vi "test-SyncMessageInCSMF.vi"(8 "error in (no error)":errorcluster, 11 "TestCase in":refnum<class "testcase-CSMSyncMessage.lvclass">) -> (0 "error out":errorcluster, 3 "TestCase out":refnum<class "testcase-CSMSyncMessage.lvclass">)   [LabVIEW 2017, in "testcase-CSMSyncMessage.lvclass"]
uses:
  testcase-CSMSyncMessage.lvclass
  src/user.lib/_NEVSTOP/Communicable State Machine(CSM)/AdvanceAPI/CSM - Make String Arguments Safe.vi
  src/user.lib/_NEVSTOP/Communicable State Machine(CSM)/AdvanceAPI/CSM - Keywords.vi
  CSM/Global-TestcaseCSM.vi
  <vilib>/addons/_JKI Toolkits/VI Tester/TestCase.llb/TestCase.lvclass
  src/user.lib/_NEVSTOP/Communicable State Machine(CSM)/Communicable State Machine.lvlib
  C:/Program Files (x86)/National Instruments/LabVIEW 2017/vi.lib/addons/_JKI Toolkits/VI Tester/TestCase.llb/TestCase.lvclass
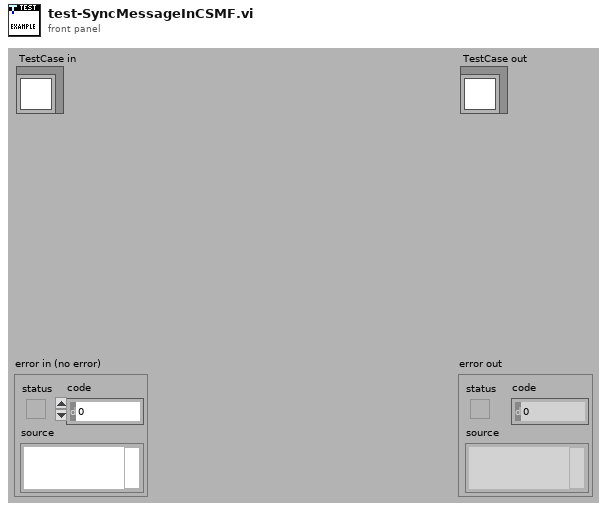
[diagram p1: front panel]
types:
  T1 = cluster{"Arguments":string, "Response":string, "error":errorcluster}
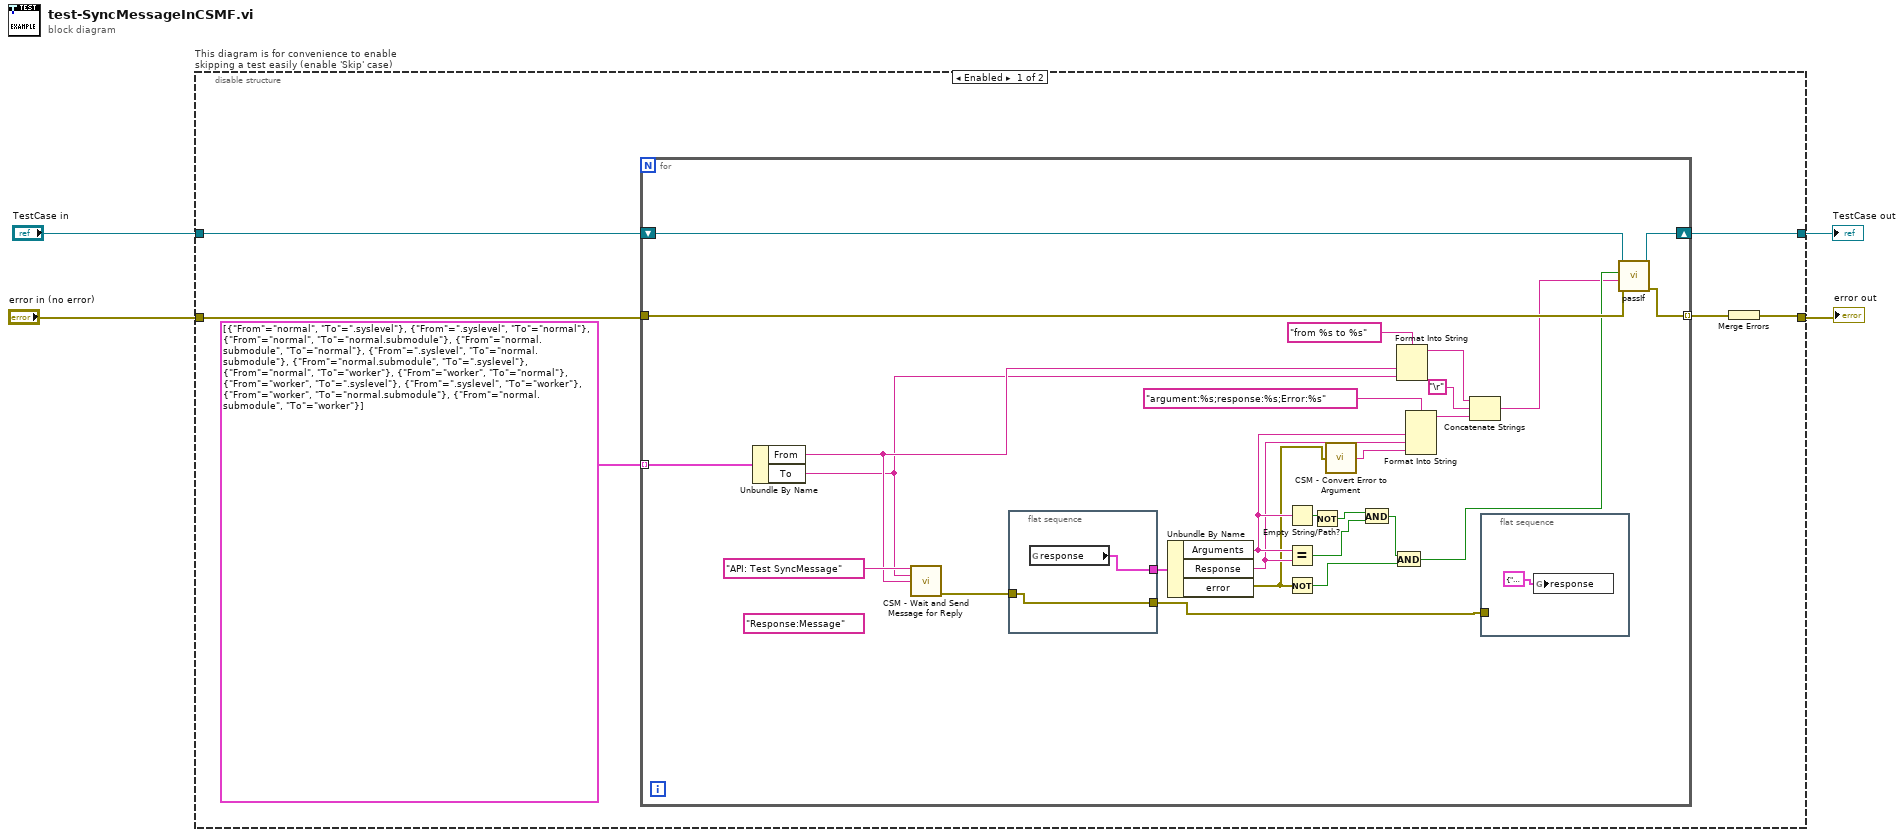
[diagram p0: block diagram]
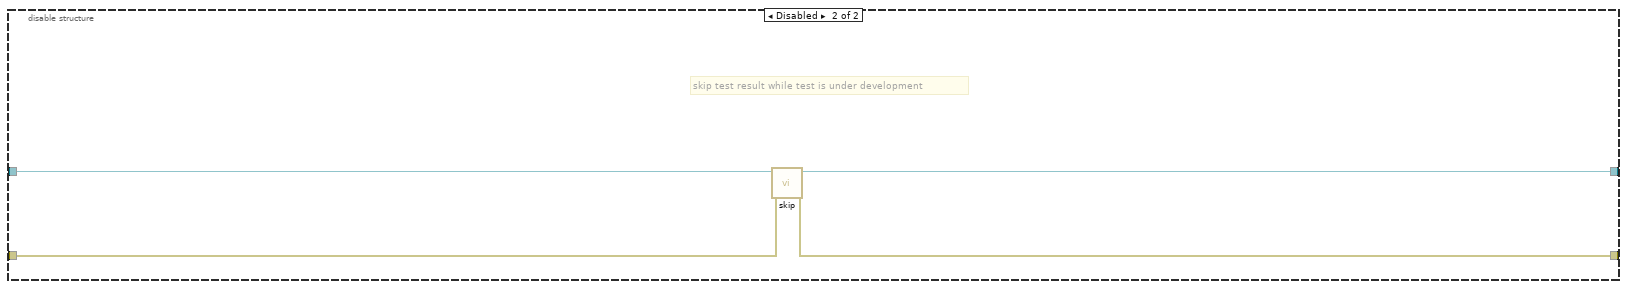
[diagram p2: hidden frame]
diagram:
  n1 = disable-structure "This diagram is for convenience to enable skipping a test easily (enable 'Skip' case)" shown="Enabled" {
    disable-tunnel: "TestCase in" -> [w10 w44]
    disable-tunnel: [w9 w42] -> w1
    disable-tunnel: [w6 w43] -> w3
    disable-tunnel: "error in (no error)" -> [w7 w41]
    frame Enabled {
      n2 = for {
        tunnel: cluster{"From":string, "To":string}[] [{"From"="normal", "To"=".syslevel"}, {"From"=".syslevel", "To"="normal"}, {"From"="normal", "To"="normal.submodule"}, {"From"="normal.submodule", "To"="normal"}, {"From"=".syslevel", "To"="normal.submodule"}, {"From"="normal.submodule", "To"=".syslevel"}, {"From"="normal", "To"="worker"}, {"From"="worker", "To"="normal"}, {"From"="worker", "To"=".syslevel"}, {"From"=".syslevel", "To"="worker"}, {"From"="worker", "To"="normal.submodule"}, {"From"="normal.submodule", "To"="worker"}] -> [w30] mode=indexing
        shift-right: [w36] -> w9
        shift-left: w10 -> [w37]
        tunnel: w7 -> [w34]
        tunnel: [w35] -> w8 mode=indexing
        (unwired) "Response:Message" ("State")
        n3 = Unbundle By Name(w30) -> ("From"=w29:string, "To"=w28:string)
        n4 = call "CSM - Wait and Send Message for Reply.vi"("State"="API: Test SyncMessage", "Arguments (\"\")"=w28, "Target Module"=w29) -> ("error out"=w11:errorcluster)  [unwired: 10 in, 2 out]
        n5 = flat-sequence {
          tunnel: w11 -> [w39]
          tunnel: [w40] -> w13
          tunnel: [w39] -> w12
          frame #0 {
            n6 = global read "Global-TestcaseCSM.vi" "response"() -> (w40:T1)
          }
        }
        n7 = Unbundle By Name(w13) -> ("Arguments"=w22:string, "Response"=w21:string, "error"=w19:errorcluster)
        n8 = Empty String/Path?(string/path=w22) -> (empty?=w26:bool)
        n9 = Equal?(x=w22, y=w21) -> (x = y?=w24:bool)
        n10 = Not(x=w19) -> (.not. x?=w32:bool)
        n11 = Not(x=w26) -> (.not. x?=w25:bool)
        n12 = call "CSM - Convert Error to Argument.vi"("Error"=w19) -> ("Argument"=w20:string)  [unwired: 4 in]
        n13 = And(x=w25, y=w24) -> (x .and. y?=w23:bool)
        n14 = And(x=w23, y=w32) -> (x .and. y?=w31:bool)
        n15 = Format Into String(format string="from %s to %s", w29, w28) -> (resulting string=w15:string)  [unwired: 2 in, 1 out]
        n16 = Format Into String(format string="argument:%s;response:%s;Error:%s", w22, w21, w20) -> (resulting string=w18:string)  [unwired: 2 in, 1 out]
        n17 = Concatenate Strings(w15, "\r", w18) -> (w16:string)
        n18 = flat-sequence {
          tunnel: w12 -> [_]
          frame #0 {
            n19 = global write "Global-TestcaseCSM.vi" "response"(T1 {"Arguments"="", "Response"="", "error"={"status"=FALSE, "code"=0, "source"=""}} ("response")) -> ()
          }
        }
        n20 = call-dynamic "passIf.vi"("error in (no error)"=w34, "message (\"\")"=w16, "pass"=w31, "TestCase in"=w37) -> ("error out"=w35:errorcluster, "TestCase out"=w36:refnum<class "testcase-CSMSyncMessage.lvclass">)  [unwired: 6 in]
      }
      n21 = Merge Errors(w8) -> (w6:errorcluster)
    }
    frame Disabled {
      # "skip test result while test is under development"
      n22 = call <vilib>:"skip.vi"("error in (no error)"=w41, "TestCase in"=w44) -> ("error out"=w43:errorcluster, "TestCase out"=w42:refnum<class "testcase-CSMSyncMessage.lvclass">)  [unwired: 8 in]
    }
  }
  "error out" <- w3
  "TestCase out" <- w1
